vi "Capture the Project refs.vi"(8 "error in":errorcluster, 10 "Target Selection":string, 11 "Project Selection":string) -> (0 "error out":errorcluster, 3 "References":T1)   [LabVIEW 2019, in "Panther Dashboard.lvlib"]
uses:
  Panther Dashboard.lvlib
  Project References--cluster.ctl
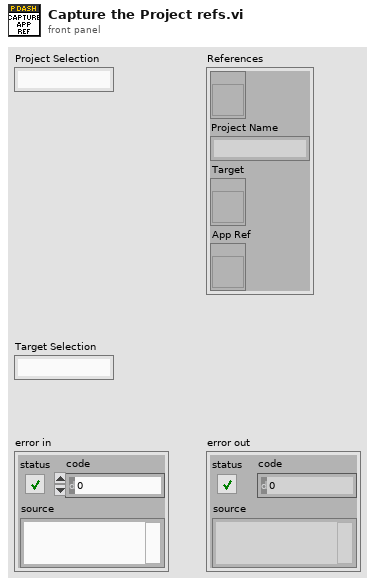
[diagram p1: front panel]
types:
  T1 = typedef "Panther Dashboard.lvlib/Project References--cluster.ctl" = cluster{"Project Ref":refnum<vi>, "Project Name":string, "Target":refnum<vi>, "App Ref":refnum<vi>}
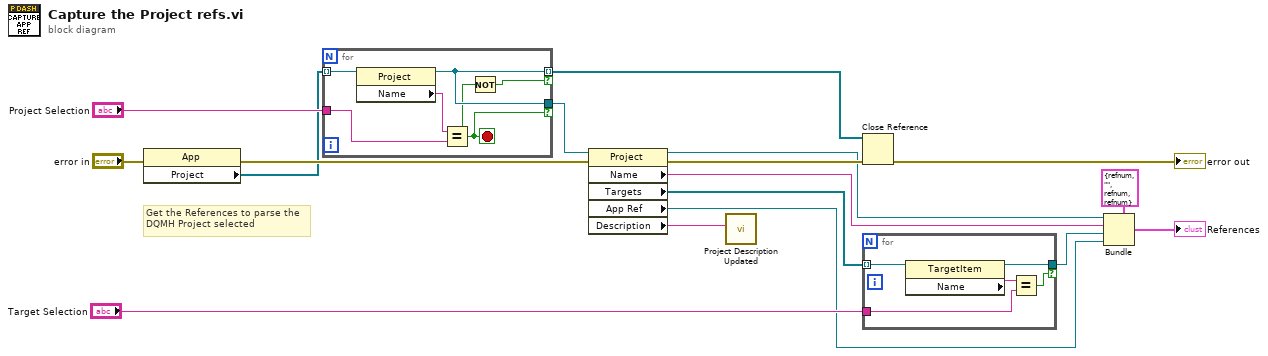
[diagram p0: block diagram]
diagram:
  # "Get the References to parse the\nDQMH Project selected"
  n1 = property class="App"(error in="error in") -> (error out=w16:errorcluster, "Project"=w7:refnum<vi>[])  [unwired: 1 in, 1 out]
  n2 = for {
    tunnel: w7 -> [w23] mode=indexing
    tunnel: [w20] -> w12 if=w19
    tunnel: "Project Selection" -> [w21]
    tunnel: [w20] -> w6 mode=indexing if=w18
    stop <- w19 stop-if-true
    n3 = property class="Project"(reference=w23) -> (reference out=w20:refnum<vi>, "Name"=w22:string)  [unwired: 1 in, 1 out]
    n4 = Equal?(x=w22, y=w21) -> (x = y?=w19:bool)
    n5 = Not(x=w19) -> (.not. x?=w18:bool)
  }
  n6 = property class="Project"(reference=w12, error in=w16) -> (reference out=w11:refnum<vi>, error out=w15:errorcluster, "Name"=w10:string, "Targets"=w5:refnum<vi>[], "App Ref"=w2:refnum<vi>, "Description"=w1:string)
  n7 = call "Project Description Updated.vi"("Project Description"=w1) -> ()  [unwired: 10 in, 1 out]
  n8 = Close Reference(reference=w6, error in (no error)=w15) -> (error out=→"error out":errorcluster)
  n9 = for {
    tunnel: w5 -> [w28] mode=indexing
    tunnel: "Target Selection" -> [w26]
    tunnel: [w25] -> w3 if=w24
    n10 = property class="TargetItem"(reference=w28) -> (reference out=w25:refnum<vi>, "Name"=w27:string)  [unwired: 1 in, 1 out]
    n11 = Equal?(x=w27, y=w26) -> (x = y?=w24:bool)
  }
  n12 = Bundle(cluster=T1 {"Project Ref"=refnum, "Project Name"="", "Target"=refnum, "App Ref"=refnum} ("References"), "Project Ref"=w11, "Project Name"=w10, "Target"=w3, "App Ref"=w2) -> (→"References":T1)
